vi "Set ROIAndBin.vi"(8 "error in (no error)":errorcluster, 9 "Region of Interest":T1={"Origin - X"=0, "Origin - Y"=0, "Width"=1392, "Height"=1040}, 10 "Binning":T2, 11 "TLCamera reference in":refnum<k24>) -> (0 "error out":errorcluster, 3 "TLCamera reference out":refnum<k24>)   [LabVIEW 2015]
uses:
  C:/code/Host/Installer/Scientific Camera Interfaces/LabVIEW/64_bit/Library_X64/Thorlabs.TSI.TLCameraInterfaces.dll
  64_bit/Library_X64/Thorlabs.TSI.TLCameraInterfaces.dll
  Controls/Binning.ctl
  Controls/Region of Interest.ctl
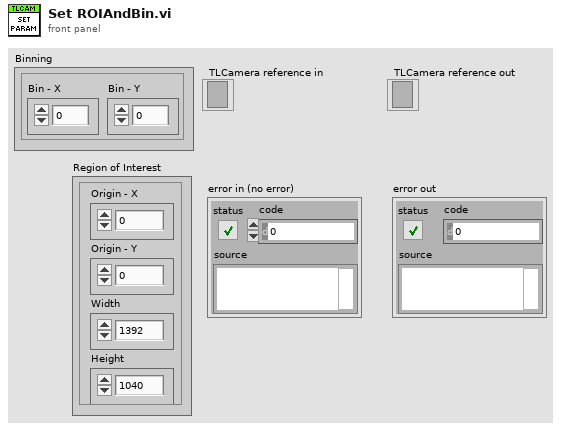
[diagram p1: front panel]
types:
  T1 = typedef "Region of Interest.ctl" = cluster{"Origin - X":u32, "Origin - Y":u32, "Width":u32, "Height":u32}
  T2 = typedef "Binning.ctl" = cluster{"Bin - X":u32, "Bin - Y":u32}
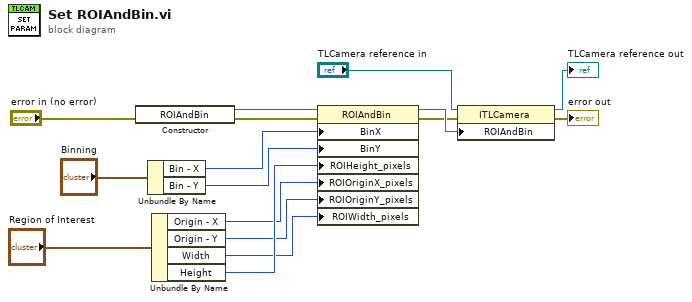
[diagram p0: block diagram]
diagram:
  n1 = constructor class="ROIAndBin"(error in="error in (no error)") -> (reference out=w14:refnum<k24>, error out=w12:errorcluster)  [unwired: 2 in, 1 out]
  n2 = Unbundle By Name("Binning") -> ("Bin - X"=w9:u32, "Bin - Y"=w8:u32)
  n3 = Unbundle By Name("Region of Interest") -> ("Origin - X"=w5:u32, "Origin - Y"=w4:u32, "Width"=w6:u32, "Height"=w7:u32)
  n4 = property class="ROIAndBin"(reference=w14, error in=w12, "BinX"=w9, "BinY"=w8, "ROIHeight_pixels"=w7, "ROIOriginX_pixels"=w5, "ROIOriginY_pixels"=w4, "ROIWidth_pixels"=w6) -> (reference out=w3:refnum<k24>, error out=w2:errorcluster)
  n5 = property class="ITLCamera"(reference="TLCamera reference in", error in=w2, "ROIAndBin"=w3) -> (reference out=→"TLCamera reference out":refnum<k24>, error out=→"error out":errorcluster)
